vi "magnitude.vi"(10 "upper limit":dbl, 11 "upper limit 2":dbl) -> (3 "Numeric":dbl)   [LabVIEW 2014]
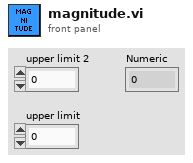
[diagram p1: front panel]
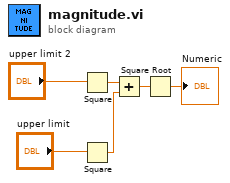
[diagram p0: block diagram]
diagram:
  n1 = Square(x="upper limit 2") -> (x^2=w1:dbl)
  n2 = Square(x="upper limit") -> (x^2=w2:dbl)
  n3 = Add(x=w1, y=w2) -> (x+y=w3:dbl)
  n4 = Square Root(x=w3) -> (sqrt(x)=→"Numeric":dbl)
